vi "setup.vi"(8 "error in (no error)":errorcluster, 11 "DAQmx_pulse_out in":refnum<class "DAQmx_DO.lvclass">) -> (0 "error out":errorcluster, 3 "DAQmx_pulse_out out":refnum<class "DAQmx_DO.lvclass">)   [LabVIEW 2013, in "DAQmx_DO.lvclass"]
uses:
  DAQmx_DO.lvclass
  DAQmx_DO.lvclass/DAQmx_DO.ctl
  <vilib>/DAQmx/write.llb/DAQmx Write (Digital Wfm 1Chan NSamp).vi
  Globals.vi
  <vilib>/DAQmx/create/channels.llb/DAQmx Create Channel (DO-Digital Output).vi
  <vilib>/DAQmx/configure/timing.llb/DAQmx Timing (Sample Clock).vi
  <vilib>/DAQmx/configure/trigger.llb/DAQmx Start Trigger (Digital Edge).vi
  <vilib>/Waveform/DWDTOps.llb/DWDT Uncompress Digital.vi
  <vilib>/DAQmx/miscellaneous.llb/DAQmx Fill In Error Info.vi
panel:
  out "output waveform":digitaldata
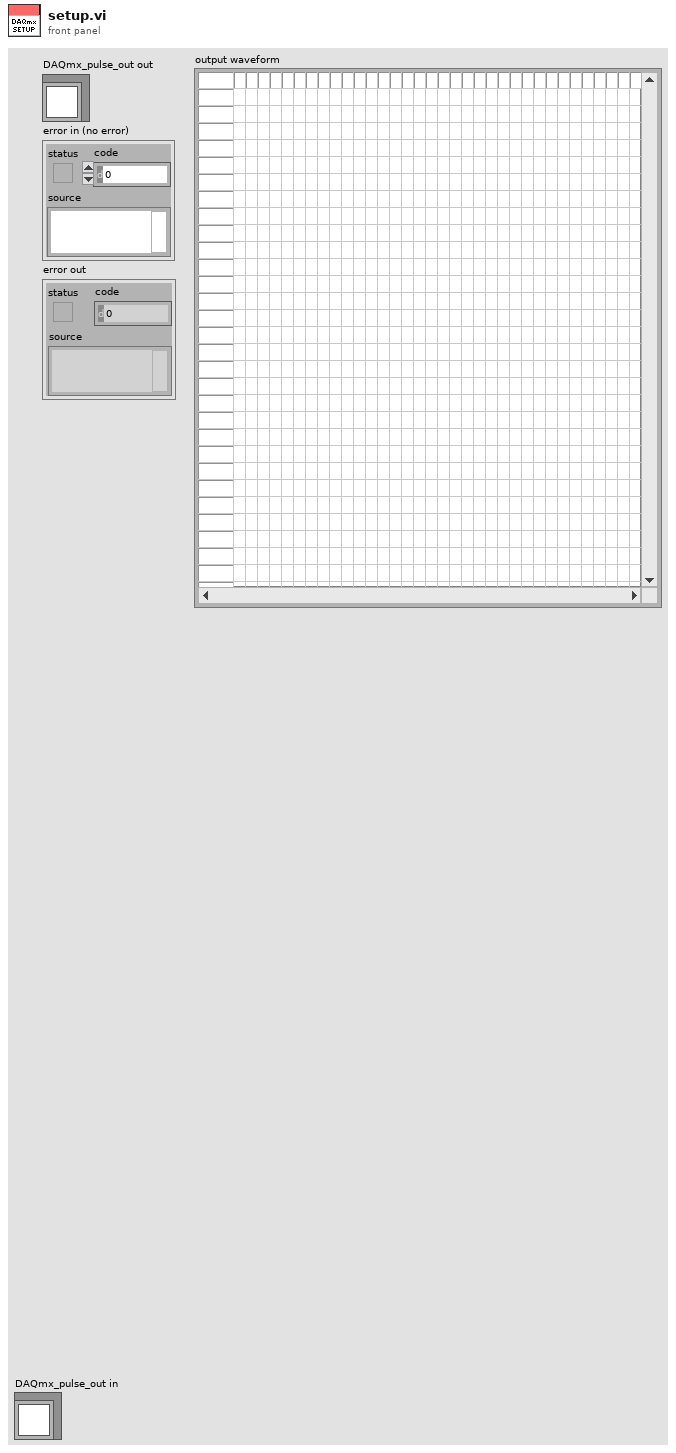
[diagram p1: front panel]
types:
  T1 = typedef "DAQmx_DO.lvclass/settings.ctl" = cluster{"Enable DAQmx Pulses":bool, "DAQmx Physical Channels":tag, "Clock Rate":dbl, "units/sec (ms=1000)":dbl, "Start Trigger":cluster{"Wait for start trigger?":bool, "source":tag, "edge":i32}, "waveform":T2}
  T2 = typedef "HSDIO.lvclass/waveform.ctl" = cluster{"name":string, "transitions":u32[], "states":u8[][]}
  T3 = cluster{"Wait for start trigger?":bool, "source":tag, "edge":i32}
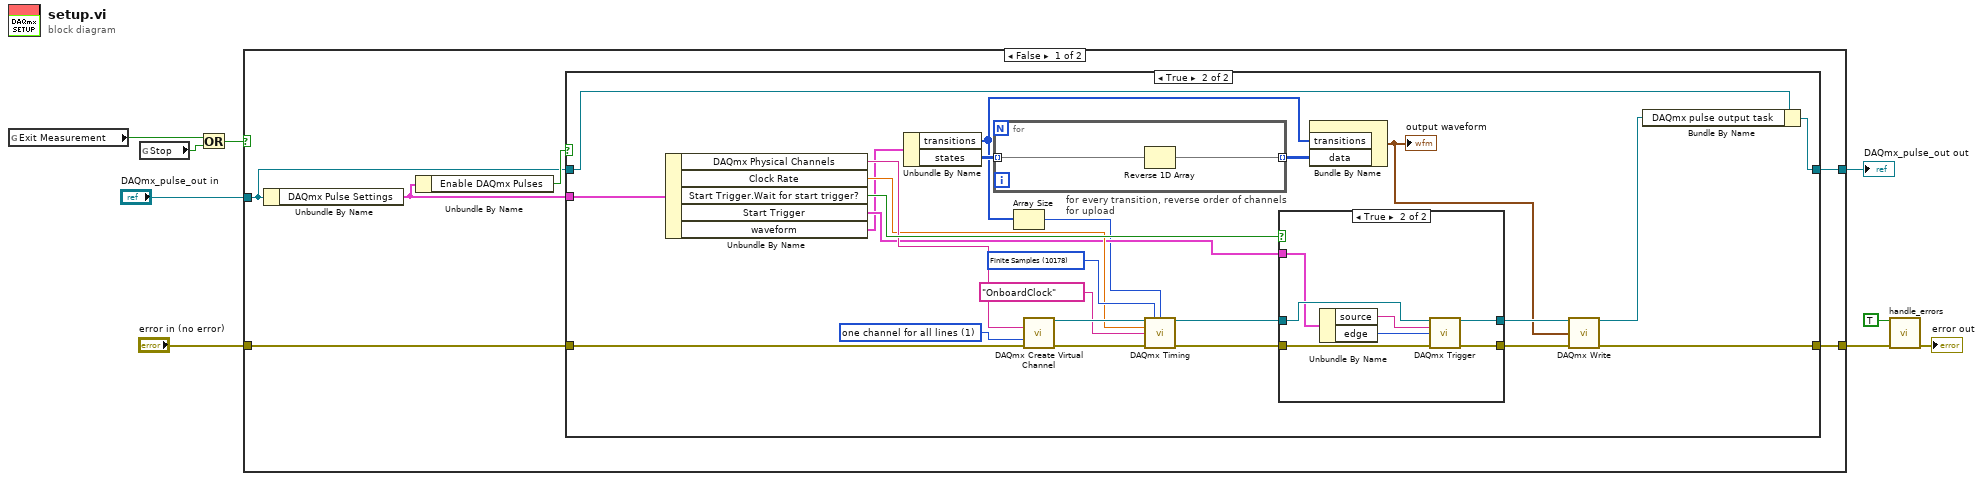
[diagram p0: block diagram]
diagram:
  n1 = global read "Globals.vi" "Exit Measurement"() -> (w6:bool)
  n2 = global read "Globals.vi" "Stop"() -> (w5:bool)
  n3 = Or(x=w6, y=w5) -> (x .or. y?=w4:bool)
  n4 = case shown="False" w4 {
    tunnel: [w14 w54] -> w3
    tunnel: [w15 w55] -> w8
    tunnel: "DAQmx_pulse_out in" -> [w11 w55]
    tunnel: "error in (no error)" -> [w12 w54]
    frame False {
      n5 = Unbundle By Name(w11) -> ("DAQmx Pulse Settings"=w10:T1)
      n6 = Unbundle By Name(w10) -> ("Enable DAQmx Pulses"=w13:bool)
      n7 = case shown="True" w13 {
        tunnel: w12 -> [w16 w26]
        tunnel: w11 -> [w17 w24]
        tunnel: [w17 w38] -> w15
        tunnel: [w16 w37] -> w14
        tunnel: w10 -> [_ w23]
        frame False {
        }
        frame True {
          w29 = 1 items=["one channel for each line", "one channel for all lines"] ("line grouping")
          w40 = 10178 items=["Finite Samples"=10178, "Continuous Samples"=10123, "Hardware Timed Single Point"=12522] ("sample mode")
          n8 = Unbundle By Name(w23) -> ("DAQmx Physical Channels"=w32:tag, "Clock Rate"=w31:dbl, "Start Trigger.Wait for start trigger?"=w33:bool, "Start Trigger"=w30:T3, "waveform"=w21:T2)
          n9 = Unbundle By Name(w21) -> ("transitions"=w18:u32[], "states"=w19:u8[][])
          n10 = for "for every transition, reverse order of channels for upload" {
            tunnel: w19 -> [w44] mode=indexing
            tunnel: [w43] -> w20 mode=indexing
            n11 = Reverse 1D Array(array=w44) -> (reversed array=w43:u8[])
          }
          n12 = Array Size(array=w18) -> (size(s)=w25:i32)
          n13 = call-poly <vilib>:"DAQmx Create Virtual Channel.vi"("lines"=w32, "line grouping"=w29, "error in"=w26) -> ("task out"=w42:refnum<k21>, "error out"=w41:errorcluster)  [unwired: 11 in]
          n14 = call-poly <vilib>:"DAQmx Timing.vi"("task/channels in"=w42, "sample mode"=w40, "samples per channel"=w25, "rate"=w31, "source"=tag "OnboardClock", "error in"=w41) -> ("task out"=w36:refnum<k21>, "error out"=w34:errorcluster)  [unwired: 8 in]
          n15 = case shown="True" w33 {
            tunnel: w36 -> [w46 w53]
            tunnel: [w46 w52] -> w35
            tunnel: w34 -> [w45 w51]
            tunnel: w30 -> [_ w50]
            tunnel: [w45 w47] -> w28
            frame False {
            }
            frame True {
              n16 = Unbundle By Name(w50) -> ("source"=w49:tag, "edge"=w48:i32)
              n17 = call-poly <vilib>:"DAQmx Trigger.vi"("task/channels in"=w53, "source"=w49, "edge"=w48, "error in"=w51) -> ("task out"=w52:refnum<k21>, "error out"=w47:errorcluster)  [unwired: 10 in]
            }
          }
          n18 = Bundle By Name("transitions"=w18, "data"=w20) -> (w22:digitaldata)  [unwired: 1 in]
          "output waveform" <- w22
          n19 = call-poly <vilib>:"DAQmx Write.vi"("task/channels in"=w35, "data"=w22, "error in"=w28) -> ("task out"=w39:refnum<k21>, "error out"=w37:errorcluster)  [unwired: 10 in, 1 out]
          n20 = Bundle By Name(cluster=w24, "DAQmx pulse output task"=w39) -> (w38:refnum<class "DAQmx_DO.lvclass">)
        }
      }
    }
    frame True {
    }
  }
  "DAQmx_pulse_out out" <- w8
  n21 = call "handle_errors.vi"("Exit Operation"=TRUE, "error in (no error)"=w3) -> ("error out"=→"error out":errorcluster)  [unwired: 13 in]
